vi "Get Test Config File Path.vi"(8 "error in (no error)":errorcluster, 11 "Base Class Test in":refnum<class "Base Test.lvclass">) -> (0 "error out":errorcluster, 2 "Test config path":path, 3 "Base Class Test out":refnum<class "Base Test.lvclass">)   [LabVIEW 2020, in "Base Test.lvclass"]
uses:
  Base Test.lvclass
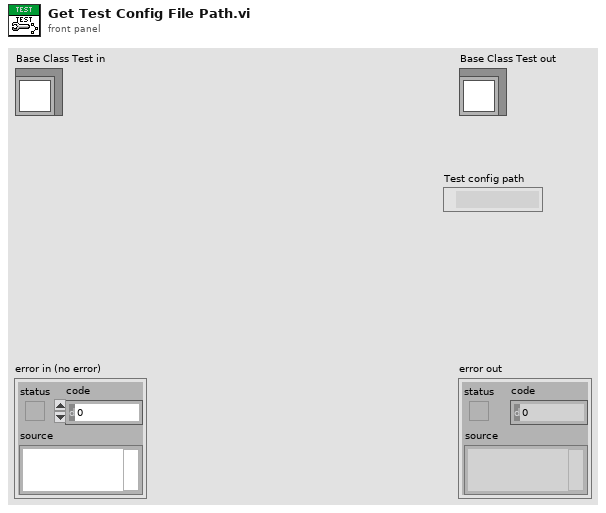
[diagram p1: front panel]
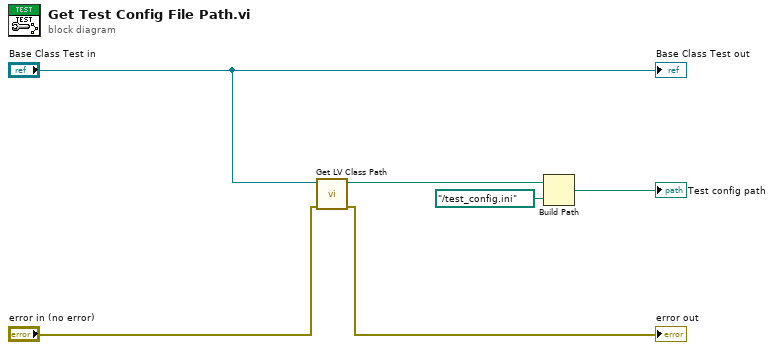
[diagram p0: block diagram]
diagram:
  n1 = call <vilib>:"Get LV Class Path.vi"("error in (no error)"="error in (no error)", "object"="Base Class Test in") -> ("error out"=→"error out":errorcluster, "class path"=w6:path)  [unwired: 8 in]
  n2 = Build Path(base path=w6, name or relative path=path "../test_config.ini") -> (appended path=→"Test config path":path)
  "Base Class Test out" <- "Base Class Test in"
